vi "Start Logger.vi"(8 "error in (no error)":errorcluster, 11 "Measure Controller in":refnum<class "Process Controller.lvclass">) -> (0 "error out":errorcluster, 2 "File Path":path, 3 "Measure Controller out":refnum<class "Process Controller.lvclass">)   [LabVIEW 2016, in "Process Controller.lvclass"]
uses:
  Process Controller.lvclass
  Process Controller.lvclass/Process Controller.ctl
  Sequence Elements/Sequence Element/Sequence Element.lvclass
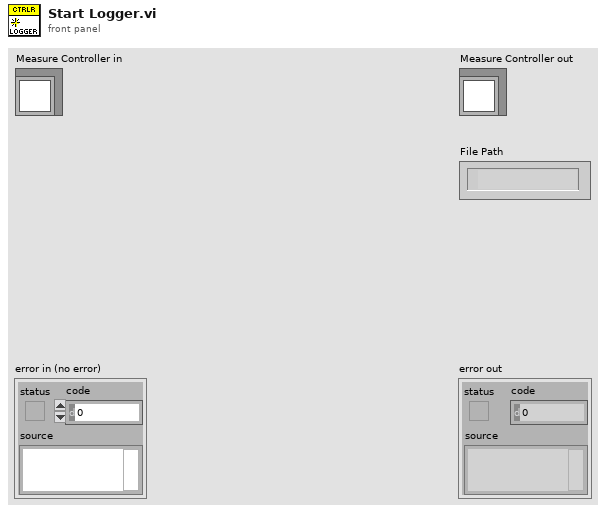
[diagram p1: front panel]
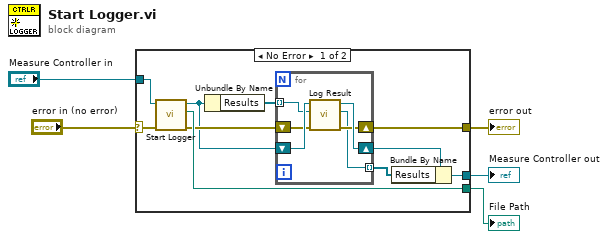
[diagram p0: block diagram]
diagram:
  n1 = case shown="No Error" "error in (no error)" {
    selector: "error in (no error)" -> [w10 w23]
    tunnel: [w12 w23] -> w4
    tunnel: [w14 w22] -> w2
    tunnel: "Measure Controller in" -> [w15 w22]
    tunnel: [w9 _] -> w1
    frame No Error {
      n2 = call-parent "Start Logger.vi"("error in (no error)"=w10, "Worker in"=w15) -> ("error out"=w8:errorcluster, "File Path"=w9:path, "Worker out"=w7:refnum<class "Process Controller.lvclass">)  [unwired: 7 in]
      n3 = Unbundle By Name(w7) -> ("Results"=w11:refnum<class "Acquired Result.lvclass">[])
      n4 = for {
        tunnel: w11 -> [w19] mode=indexing
        shift-right: [w17] -> w12
        shift-left: w8 -> [w18]
        tunnel: [w16] -> w13 mode=indexing
        shift-right: [w20] -> w6
        shift-left: w7 -> [w21]
        n5 = call-dynamic "Log Result.vi"("error in (no error)"=w18, "Result"=w19, "Process Controller in"=w21) -> ("error out"=w17:errorcluster, "Result out"=w16:refnum<class "Acquired Result.lvclass">, "Process Controller out"=w20:refnum<class "Process Controller.lvclass">)  [unwired: 6 in]
      }
      n6 = Bundle By Name(cluster=w6, "Results"=w13) -> (w14:refnum<class "Process Controller.lvclass">)
    }
    frame Error {
    }
  }
  "error out" <- w4
  "Measure Controller out" <- w2
  "File Path" <- w1
